vi "Performance test.vi"() -> ()   [LabVIEW 2012]
panel:
  in  "DCborderWidth":i32
  in  "useLUT":bool
  in  "Use polynomial \nLUT":bool
  in  "Polynomial Order":i32=3 min=3 max=7 step=1
  in  "Save\nAmplitudes":bool
  in  "Aberration \nCorrection On":bool
  in  "deviceId":i32
  in  "Path to LUT file":path=path "C:/BLINK_PCIe/LUT_Files/linear.lut"
  out "XY Graph":cluster{i32[], dbl[]}(graph)={[1, 2], [4.621621621621622, 5.528528528528528]}
  out "Last number \nof spots":i32=1
  out "Last execution \ntime":dbl=5.528528528528528
  in  "alpha RPC":sgl=1.0
  in  "Number of spotsmax":i32=100
  in  "Number of spots min":i32=1
  in  "TrueFrame":i32=3
  in  "Number of \ntime to execute":i32=100
  in  "stop program":bool
  out "Generated Hologram":u8[][](graph)
  in  "Method":i32(ring)=1 items=["Lenses & Gratings (3D)", "Gerschberg-Saxton Fresnel (3D)", "Gerschberg-Saxton FFT (2D)"]
  in  "N_iterations":i32=10
  in  "SLM enabled":bool
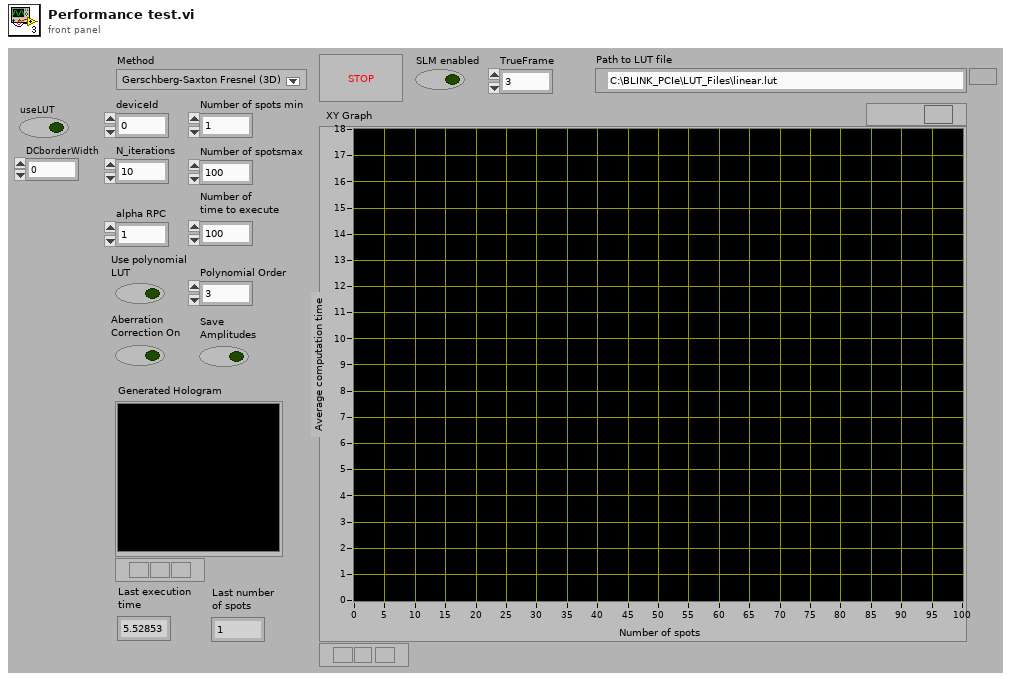
[diagram p1: front panel]
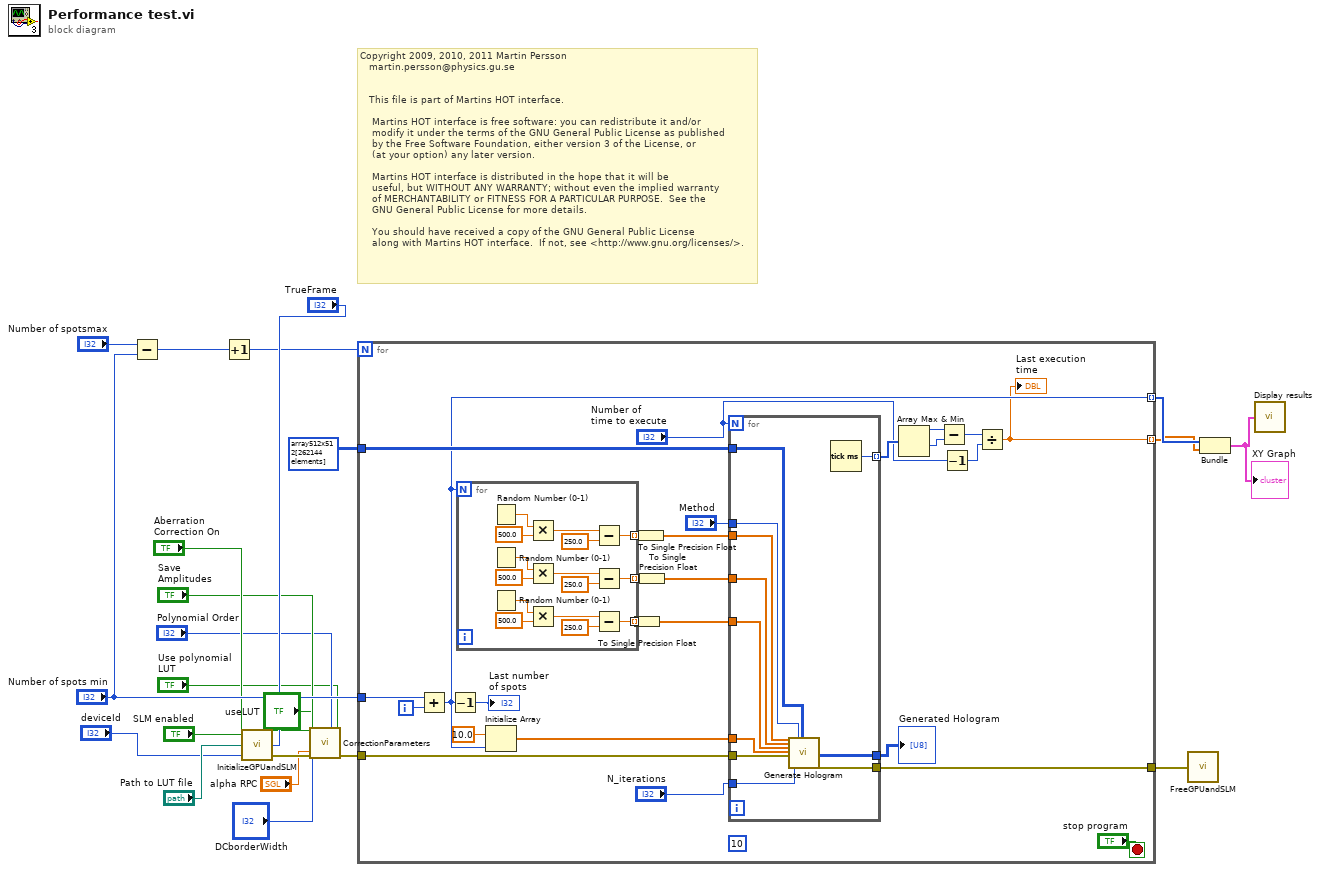
[diagram p0: block diagram]
diagram:
  # "Copyright 2009, 2010, 2011 Martin Persson \n   martin.persson@physics.gu.se\n\n\n   This file is part of Martins HOT interface.\n\n    Martins HOT interface is free software: you can redistribute it and/or \n    modify it under the terms of the GNU General Public License as published \n    by the Free Software Foundation, either version 3 of the License, or\n    (at your option) any later version.\n\n    Martins HOT interface is distributed in the hope that it will be \n    useful, but WITHOUT ANY WARRANTY; without even the implied warranty\n    of MERCHANTABILITY or FITNESS FOR A PARTICULAR PURPOSE.  See the\n    GNU General Public License for more details.\n\n    You should have received a copy of the GNU General Public License\n    along with Martins HOT interface.  If not, see <http://www.gnu.org/licenses/>."
  n1 = Subtract(x="Number of spotsmax", y="Number of spots min") -> (x-y=w18:i32)
  n2 = Increment(x=w18) -> (x+1=w16:i32)
  n3 = call "InitializeGPUandSLM.vi"("TrueFrame"="TrueFrame", "deviceId"="deviceId", "Path to LUT file"="Path to LUT file", "SLM enabled"="SLM enabled") -> ("CUDA/SLM error"=w9:errorcluster)  [unwired: 1 out]
  n4 = call "CorrectionParameters.vi"("Aberration Correction On"="Aberration \nCorrection On", "Polynomial Order"="Polynomial Order", "SaveAmplitudes"="Save\nAmplitudes", "useLUT"="useLUT", "DCborderWidth"="DCborderWidth", "Use polynomial LUT"="Use polynomial \nLUT", "error in"=w9, "AlphaRPC"="alpha RPC") -> ("error out"=w8:errorcluster)  [unwired: 6 in, 1 out]
  n5 = for {
    N: w16 -> [_]
    tunnel: w8 -> [w48]
    tunnel: [w45] -> w21
    tunnel: u8[][] array512x512[262144 elements] ("Default") -> [w43]
    tunnel: "Number of spots min" -> [w35]
    tunnel: [w28] -> w12 mode=indexing
    tunnel: [w29] -> w13 mode=indexing
    i -> [w34]
    stop <- "stop program" stop-if-true
    (unwired) 10 ("element")
    n6 = Add(x=w35, y=w34) -> (x+y=w29:i32)
    n7 = Decrement(x=w29) -> (x-1=→"Last number \nof spots":i32)
    n8 = for {
      N: w29 -> [_]
      tunnel: [w52] -> w33 mode=indexing
      tunnel: [w51] -> w32 mode=indexing
      tunnel: [w50] -> w31 mode=indexing
      n9 = Random Number (0-1)() -> (number: 0 to 1=w63:dbl)
      n10 = Random Number (0-1)() -> (number: 0 to 1=w56:dbl)
      n11 = Random Number (0-1)() -> (number: 0 to 1=w49:dbl)
      n12 = Multiply(x=w63, y=500.0) -> (x*y=w61:dbl)
      n13 = Multiply(x=w56, y=500.0) -> (x*y=w58:dbl)
      n14 = Multiply(x=w49, y=500.0) -> (x*y=w54:dbl)
      n15 = Subtract(x=w61, y=250.0) -> (x-y=w52:dbl)
      n16 = Subtract(x=w58, y=250.0) -> (x-y=w51:dbl)
      n17 = Subtract(x=w54, y=250.0) -> (x-y=w50:dbl)
    }
    n18 = Initialize Array(sgl 10.0 ("element"), w29) -> (w41:sgl[])
    n19 = To Single Precision Float(number=w31) -> (single precision float=w24:sgl[])
    n20 = To Single Precision Float(number=w33) -> (single precision float=w26:sgl[])
    n21 = To Single Precision Float(number=w32) -> (single precision float=w25:sgl[])
    n22 = for {
      N: "Number of \ntime to execute" -> [_]
      tunnel: w48 -> [w74]
      tunnel: "N_iterations" -> [w73]
      tunnel: w25 -> [w72]
      tunnel: w24 -> [w71]
      tunnel: "Method" -> [w70]
      tunnel: [w69] -> w45
      tunnel: [w68] -> w44
      tunnel: w43 -> [w67]
      tunnel: w26 -> [w66]
      tunnel: w41 -> [w65]
      tunnel: [w64] -> w40 mode=indexing
      n23 = call "Generate Hologram.vi"("x"=w66, "y"=w72, "z"=w71, "spot_intensities"=w65, "CUDA/SLM error in"=w74, "N_iterations"=w73, "method"=w70, "CGH in"=w67) -> ("CGH out"=w68:u8[][], "CUDA/SLM error out"=w69:errorcluster)  [unwired: 16 in, 2 out]
      n24 = Tick Count (ms)() -> (millisecond timer value=w64:u32)
    }
    "Generated Hologram" <- w44
    n25 = Array Max & Min(array=w40) -> (max value=w39:u32, min value=w38:u32)  [unwired: 2 out]
    n26 = Subtract(x=w39, y=w38) -> (x-y=w37:u32)
    n27 = Decrement(x="Number of \ntime to execute") -> (x-1=w27:i32)
    n28 = Divide(x=w37, y=w27) -> (x/y=w28:dbl)
    "Last execution \ntime" <- w28
  }
  n29 = call "FreeGPUandSLM.vi"("error in"=w21) -> ()  [unwired: 2 out]
  n30 = Bundle(w13, w12) -> (w11:cluster{i32[], dbl[]})  [unwired: 1 in]
  "XY Graph" <- w11
  n31 = call "Display results.vi"("Cluster"=w11) -> ()
